vi "Configure Coupling.vi"(8 "error in (no error)":errorcluster, 9 "Vertical Coupling (0: A1M)":u16(ring) items=["A1M", "D1M", "D50", "Ground", "DC", "AC"], 10 "Channel (0: Channel 1)":u16(ring) items=["Channel 1", "Channel 2", "Channel 3", "Channel 4", "EX", "EX10"], 11 "VISA resource name":refnum<visa-resource-name>) -> (0 "error out":errorcluster, 3 "VISA resource name out":refnum<visa-resource-name>)   [LabVIEW 2013, in "LeCroy Wave Series.lvlib"]
doc: "Specify how you want the oscilloscope to couple the input signal for the channel."
uses:
  LeCroy Wave Series.lvlib
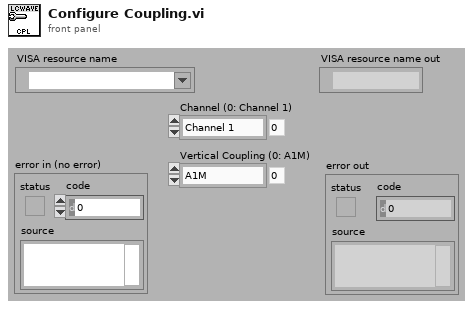
[diagram p1: front panel]
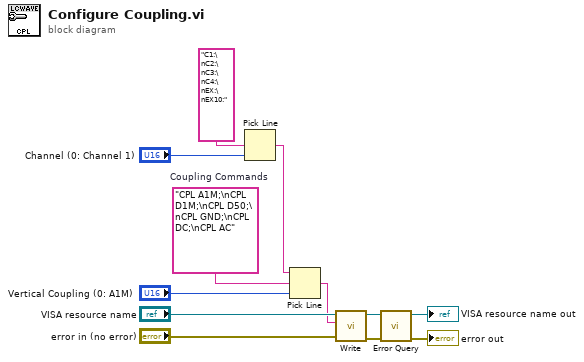
[diagram p0: block diagram]
diagram:
  w10 = "CPL A1M;\nCPL D1M;\nCPL D50;\nCPL GND;\nCPL DC;\nCPL AC"  # Coupling Commands
  n1 = Pick Line(multi-line string="C1:\nC2:\nC3:\nC4:\nEX:\nEX10:", line index="Channel (0: Channel 1)") -> (output string=w8:string)  [unwired: 1 in]
  n2 = Pick Line(string ("")=w8, multi-line string=w10, line index="Vertical Coupling (0: A1M)") -> (output string=w5:string)
  n3 = call "Write.vi"("error in (no error)"="error in (no error)", "Write Buffer"=w5, "VISA resource name"="VISA resource name") -> ("error out"=w1:errorcluster, "VISA resource name out"=w2:refnum<visa-resource-name>)  [unwired: 6 in, 1 out]
  n4 = call "Error Query.vi"("error in (no error)"=w1, "VISA resource name"=w2) -> ("error out"=→"error out":errorcluster, "VISA resource name out"=→"VISA resource name out":refnum<visa-resource-name>)  [unwired: 6 in, 2 out]
